vi "template.free.vi"(8 "error in":errorcluster, 11 "Template in":refnum<class "Template.lvclass">) -> (0 "error out":errorcluster, 3 "Template out":refnum<class "Template.lvclass">)   [LabVIEW 2020, in "Template.lvclass"]
doc: "Releases the handle and its associated resources."
uses:
  Template.lvclass
  Template.lvclass/Template.ctl
  client.lvlib
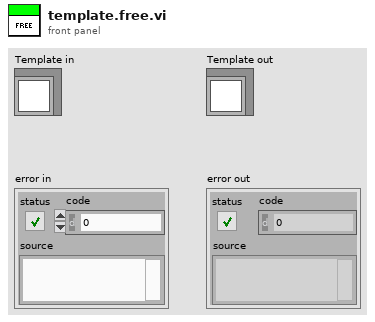
[diagram p1: front panel]
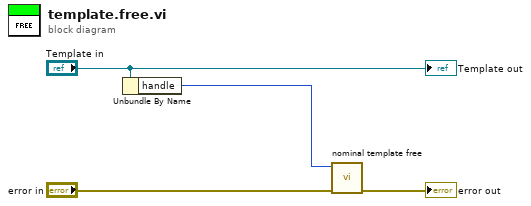
[diagram p0: block diagram]
diagram:
  n1 = Unbundle By Name("Template in") -> ("handle"=w2:i32)
  n2 = call "nominal template free.vi"("error in (no error)"="error in", "template_"=w2) -> ("error out"=→"error out":errorcluster)  [unwired: 8 in, 1 out]
  "Template out" <- "Template in"
